vi "TDS_LoadConfiguration.vi"(7 "instrument handle":refnum<k15>, 8 "error in":errorcluster, 11 "VI Server ClusterDUP":T1) -> (0 "error out":errorcluster)   [LabVIEW 2020]
uses:
  LabVIEW 2020 Toolkits/VI Server Toolkit/VI Server_TypeDefs/VI Server_RefsCluster.ctl
  LabVIEW 2020 Toolkits/VI Server Toolkit/VI Server Libraries/VI Server_GetControl.llb/VI Server_PATH_Get.vi
  LabVIEW 2020 Toolkits/VI Server Toolkit/VI Server Libraries/VI Server_Set Controls.llb/Set PATH Control.vi
  <vilib>/Utility/config.llb/Read Key (String).vi
  LabVIEW 2020 Toolkits/VI Server Toolkit/VI Server Toolkit LV2013.lvlib
  <vilib>/Utility/config.llb/NI_LVConfig.lvlib
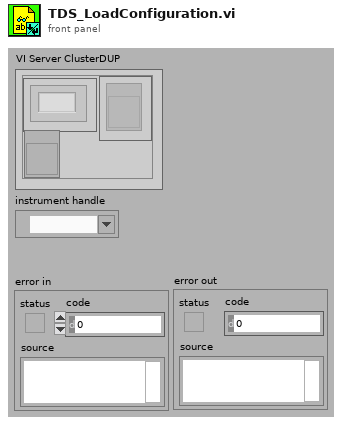
[diagram p1: front panel]
types:
  T1 = typedef "VI Server_RefsCluster.ctl" = cluster{"Labels":string[], "Refs":refnum<vi>[], "VI Ref":refnum<vi>}
  T2 = typedef "NI_LVConfig.lvlib/Config Data RefNum.ctl" = refnum<k1>
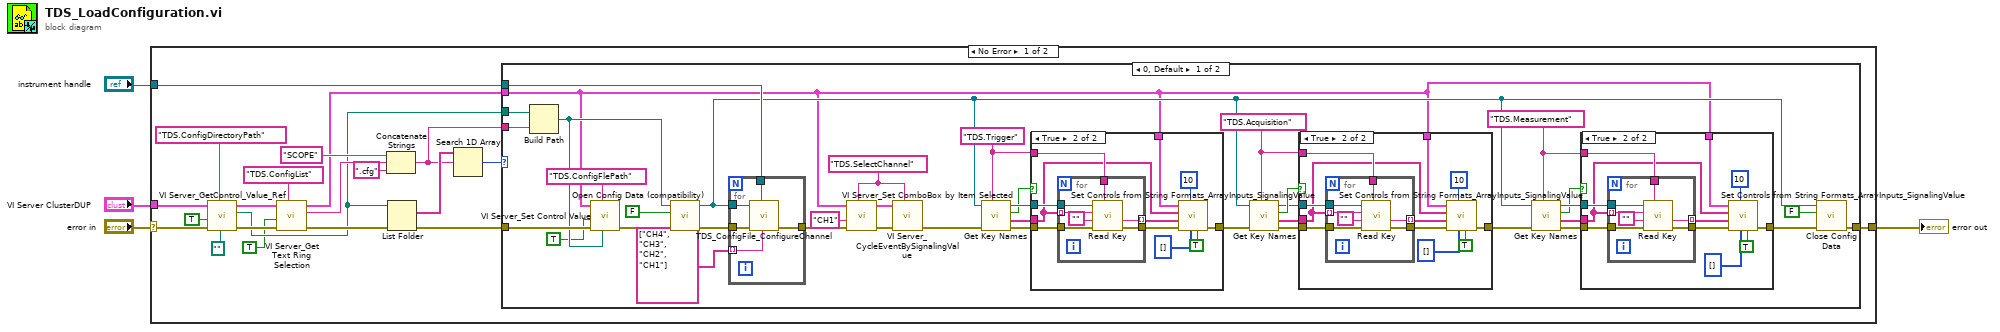
[diagram p0: block diagram]
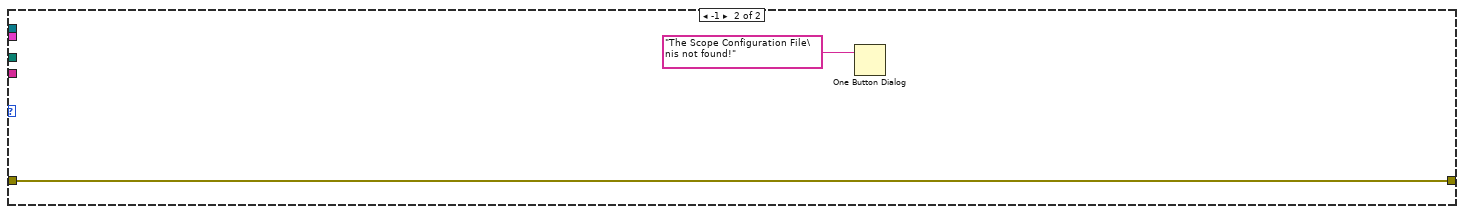
[diagram p5: hidden frame]
diagram:
  n1 = case shown="No Error" "error in" {
    selector: "error in" -> [w11 w129]
    tunnel: "VI Server ClusterDUP" -> [w13 _]
    tunnel: [w18 w129] -> w3
    tunnel: "instrument handle" -> [w14 _]
    frame No Error {
      n2 = call-poly "VI Server_GetControl_Value_Ref.vi"("DataType"=path "", "Control.Label"="TDS.ConfigDirectoryPath" ("Label"), "error in"=w11, "SingleInstance"=TRUE, "VI Server.RefsCluster"=w13) -> ("error out"=w10:errorcluster, "Value"=w8:path, "VI Server.RefsCluster.DUP"=w12:T1)  [unwired: 3 in, 1 out]
      n3 = call "VI Server_Get Text Ring Selection.vi"("Label"="TDS.ConfigList", "error in"=w10, "Single Instance (T)"=TRUE, "VI Server Cluster"=w12) -> ("error out"=w24:errorcluster, "Selection"=w21:string, "VI Server Custer.DUP"=w15:T1)  [unwired: 2 in, 3 out]
      n4 = Concatenate Strings("SCOPE" ("regular expression"), w21, ".cfg" ("string")) -> (w16:string)
      n5 = List Folder(path=w8, error in=w24) -> (filenames=w25:string[], error out=w19:errorcluster)  [unwired: 2 in, 2 out]
      n6 = Search 1D Array(1D array=w25, element=w16) -> (index of element=w17:i32)  [unwired: 1 in]
      n7 = case shown="0, Default" w17 {
        tunnel: w19 -> [w43 w128]
        tunnel: [w62 w128] -> w18
        tunnel: w16 -> [w64 _]
        tunnel: w8 -> [w63 _]
        tunnel: w15 -> [w29 _]
        tunnel: w14 -> [w53 _]
        frame 0, Default {
          w33 = "TDS.Measurement" ("section")
          w47 = "TDS.Acquisition" ("section")
          w39 = "TDS.SelectChannel" ("Label")
          w58 = "TDS.Trigger" ("section")
          n8 = Build Path(base path=w63, name or relative path=w64) -> (appended path=w40:path)
          n9 = call-poly "VI Server_Set Control Value.vi"("New Value"=w40, "Label"="TDS.ConfigFlePath", "error in"=w43, "Single Instance (T)"=TRUE, "VI Server Cluster"=w29) -> ("error out"=w42:errorcluster)  [unwired: 4 in, 2 out]
          n10 = call <vilib>:"Open Config Data (compatibility).vi"("error in (no error)"=w42, "create file if necessary (T)"=FALSE ("create file if necessary? (T)"), "configuration file path"=w40) -> ("error out"=w54:errorcluster, "refnum"=w30:T2)  [unwired: 6 in, 1 out]
          n11 = for {
            tunnel: w30 -> [w106]
            tunnel: w54 -> [w107]
            tunnel: w53 -> [w105]
            tunnel: [w104] -> w51
            tunnel: string[] ["CH4", "CH3", "CH2", "CH1"] -> [w103] mode=indexing
            n12 = call "TDS_ConfigFile_ConfigureChannel.vi"("ScopeChannel"=w103, "instrument handle"=w105, "error in"=w107, "refnum"=w106) -> ("error out"=w104:errorcluster)  [unwired: 7 in]
          }
          n13 = call "VI Server_Set ComboBox by Item Selected.vi"("Label"=w39, "error in"=w51, "Item Selected"="CH1" ("ComboBoxValue"), "VI Server Cluster"=w29) -> ("error out"=w38:errorcluster, "VI Server Cluster.DUP"=w36:T1)  [unwired: 5 in, 1 out]
          n14 = call "VI Server_CycleEventBySignalingValue.vi"("Label"=w39, "error in"=w38, "VI Server.RefsCluster"=w36) -> ("error out"=w37:errorcluster)  [unwired: 7 in, 1 out]
          n15 = call <vilib>:"Get Key Names.vi"("section"=w58, "error in (no error)"=w37, "refnum"=w30) -> ("error out"=w60:errorcluster, "key names"=w57:string[], "section exists?"=w56:bool, "refnum out"=w59:T2)  [unwired: 5 in]
          n16 = case shown="True" w56 {
            tunnel: w60 -> [w108 w119]
            tunnel: w59 -> [_ w118]
            tunnel: w58 -> [_ w117]
            tunnel: w57 -> [_ w116]
            tunnel: [w108 w113] -> w44
            tunnel: w29 -> [_ w112]
            frame False {
            }
            frame True {
              n17 = for {
                tunnel: w119 -> [w126]
                tunnel: [w125] -> w114
                tunnel: w118 -> [w124]
                tunnel: w117 -> [w123]
                tunnel: w116 -> [w122] mode=indexing
                tunnel: [w120] -> w115 mode=indexing
                n18 = call-poly <vilib>:"Read Key.vi"("section"=w123, "error in (no error)"=w126, "default value"="", "key"=w122, "refnum"=w124) -> ("error out"=w125:errorcluster, "value"=w120:string)  [unwired: 3 in, 2 out]
              }
              n19 = call "Set Controls from String Formats_ArrayInputs_SignalingValue.vi"("Defer Panel Updates (T)"=TRUE, "Disabled"=u8[] [], "milliseconds to wait (10 ms)"=u32 10, "error in (no error)"=w114, "Values"=w115, "Labels"=w116, "VI Server Cluster"=w112) -> ("error out"=w113:errorcluster)  [unwired: 3 in, 1 out]
            }
          }
          n20 = call <vilib>:"Get Key Names.vi"("section"=w47, "error in (no error)"=w44, "refnum"=w30) -> ("error out"=w45:errorcluster, "key names"=w48:string[], "section exists?"=w49:bool, "refnum out"=w46:T2)  [unwired: 5 in]
          n21 = case shown="True" w49 {
            tunnel: w45 -> [w84 w95]
            tunnel: w46 -> [_ w94]
            tunnel: w47 -> [_ w93]
            tunnel: w48 -> [_ w92]
            tunnel: [w84 w89] -> w27
            tunnel: w29 -> [_ w88]
            frame False {
            }
            frame True {
              n22 = for {
                tunnel: w95 -> [w102]
                tunnel: [w101] -> w90
                tunnel: w94 -> [w100]
                tunnel: w93 -> [w99]
                tunnel: w92 -> [w98] mode=indexing
                tunnel: [w96] -> w91 mode=indexing
                n23 = call-poly <vilib>:"Read Key.vi"("section"=w99, "error in (no error)"=w102, "default value"="", "key"=w98, "refnum"=w100) -> ("error out"=w101:errorcluster, "value"=w96:string)  [unwired: 3 in, 2 out]
              }
              n24 = call "Set Controls from String Formats_ArrayInputs_SignalingValue.vi"("Defer Panel Updates (T)"=TRUE, "Disabled"=u8[] [], "milliseconds to wait (10 ms)"=u32 10, "error in (no error)"=w90, "Values"=w91, "Labels"=w92, "VI Server Cluster"=w88) -> ("error out"=w89:errorcluster)  [unwired: 3 in, 1 out]
            }
          }
          n25 = call <vilib>:"Get Key Names.vi"("section"=w33, "error in (no error)"=w27, "refnum"=w30) -> ("error out"=w35:errorcluster, "key names"=w32:string[], "section exists?"=w31:bool, "refnum out"=w34:T2)  [unwired: 5 in]
          n26 = case shown="True" w31 {
            tunnel: w35 -> [w65 w76]
            tunnel: w34 -> [_ w75]
            tunnel: w33 -> [_ w74]
            tunnel: w32 -> [_ w73]
            tunnel: [w65 w70] -> w28
            tunnel: w29 -> [_ w69]
            frame False {
            }
            frame True {
              n27 = for {
                tunnel: w76 -> [w83]
                tunnel: [w82] -> w71
                tunnel: w75 -> [w81]
                tunnel: w74 -> [w80]
                tunnel: w73 -> [w79] mode=indexing
                tunnel: [w77] -> w72 mode=indexing
                n28 = call-poly <vilib>:"Read Key.vi"("section"=w80, "error in (no error)"=w83, "default value"="", "key"=w79, "refnum"=w81) -> ("error out"=w82:errorcluster, "value"=w77:string)  [unwired: 3 in, 2 out]
              }
              n29 = call "Set Controls from String Formats_ArrayInputs_SignalingValue.vi"("Defer Panel Updates (T)"=TRUE, "Disabled"=u8[] [], "milliseconds to wait (10 ms)"=u32 10, "error in (no error)"=w71, "Values"=w72, "Labels"=w73, "VI Server Cluster"=w69) -> ("error out"=w70:errorcluster)  [unwired: 3 in, 1 out]
            }
          }
          n30 = call <vilib>:"Close Config Data.vi"("error in (no error)"=w28, "write file if changed (T)"=FALSE ("write configuration file? (T)"), "refnum"=w30) -> ("error out"=w62:errorcluster)  [unwired: 7 in, 1 out]
        }
        frame -1 {
          n31 = One Button Dialog(message="The Scope Configuration File\nis not found!") -> ()  [unwired: 1 in, 1 out]
        }
      }
    }
    frame Error {
    }
  }
  "error out" <- w3
